vi "Update H2H Array.vi"(9 "# of Fields":i32, 10 "New Row":i32[](array[numeric]), 11 "H2H Array":i32[][](array[numeric])) -> (3 "H2H Array Out":i32[][](array[numeric]))   [LabVIEW 2013]
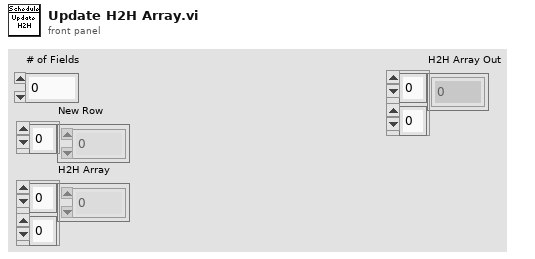
[diagram p1: front panel]
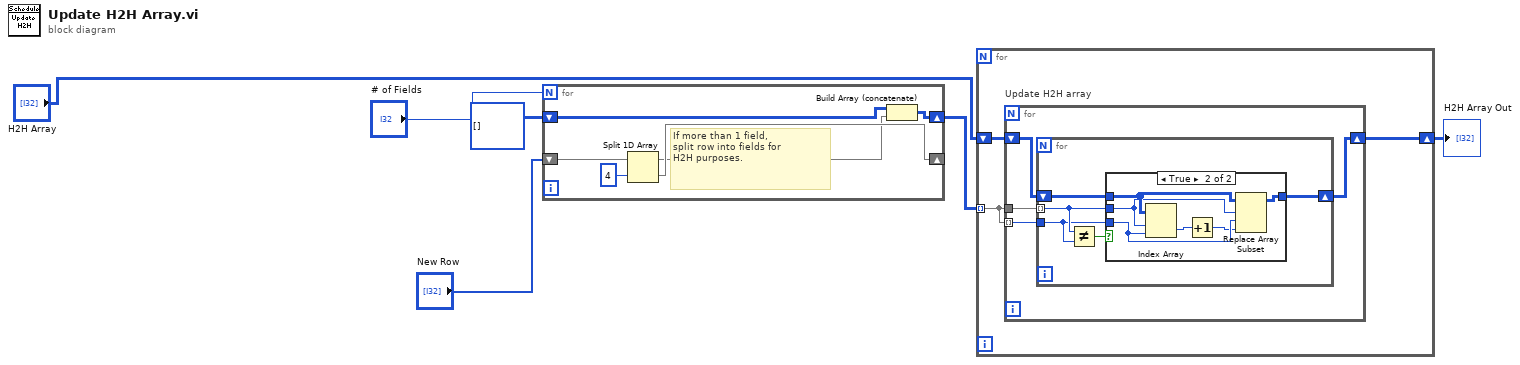
[diagram p0: block diagram]
diagram:
  n1 = for {
    N: "# of Fields" -> [_]
    shift-right: [w11] -> w5
    shift-left: i32[][] [] -> [w12]
    shift-right: [w8] -> _
    shift-left: "New Row" -> [w10]
    # "If more than 1 field, \nsplit row into fields for \nH2H purposes."
    n2 = Split 1D Array(array=w10, index=4) -> (first subarray=w7:i32[], second subarray=w8:i32[])
    n3 = Build Array (concatenate)(w12, w7) -> (w11:i32[][])
  }
  n4 = for {
    tunnel: w5 -> [w13] mode=indexing
    shift-right: [w14] -> w1
    shift-left: "H2H Array" -> [w15]
    n5 = for "Update H2H array" {
      tunnel: w13 -> [w18] mode=indexing
      tunnel: w13 -> [w19]
      shift-right: [w16] -> w14
      shift-left: w15 -> [w17]
      n6 = for {
        tunnel: w19 -> [w22] mode=indexing
        tunnel: w18 -> [w21]
        shift-right: [w20] -> w16
        shift-left: w17 -> [w23]
        n7 = Not Equal?(x=w22, y=w21) -> (x != y?=w24:bool)
        n8 = case shown="True" w24 {
          tunnel: w23 -> [w25 w31]
          tunnel: w22 -> [_ w30]
          tunnel: w21 -> [_ w29]
          tunnel: [w25 w26] -> w20
          frame False {
          }
          frame True {
            n9 = Index Array(array=w31, index (row)=w30, index (col)=w29) -> (element=w28:i32)
            n10 = Increment(x=w28) -> (x+1=w27:i32)
            n11 = Replace Array Subset(array=w31, new element=w27, index (row)=w30, index (col)=w29) -> (w26:i32[][])
          }
        }
      }
    }
  }
  "H2H Array Out" <- w1
